vi "niFPGA White Noise Generator.vi"(0 "seed":u32=4294967295, 1 "reset":bool) -> (4 "white noise out":i16)   [LabVIEW 2017]
doc: "Generates a white noise signal with uniform or Gaussian distribution."
uses:
  <vilib>/Platform/TimedLoop/XDataNode/timing_clust.ctl
  <vilib>/Platform/TimedLoop/XDataNode/nitl_modes.ctl
  <vilib>/Platform/TimedLoop/XDataNode/wakeup.ctl
  <vilib>/Platform/TimedLoop/XDataNode/XDataNode.xnode
  <vilib>/Platform/TimedLoop/XDataNode/XDNodeRunTimeDep.lvlib
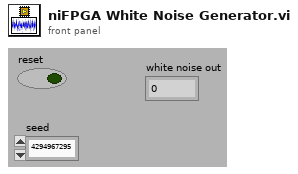
[diagram p1: front panel]
types:
  T1 = typedef "XDNodeRunTimeDep.lvlib/timing_clust.ctl" = cluster{"Expected End [f-1]":u64, "Actual End [f-1]":u64, "Finished Late? [f-1]":bool, "Expected End [i-1]":u64, "Actual End [i-1]":u64, "Finished Late? [i-1]":bool, "Expected Start [i]":u64, "Actual Start [i]":u64, "Expected Start [f]":u64, "Actual Start [f]":u64, "Source Name":string, "Structure Name":string, "Period":i64, "Deadline":i64, "Offset":i64, "Start":i64, "Priority":i32, "Timeout":i32, "Mode":T2, "Wakeup Reason":T3, "Error":errorcluster, "Source Type":string, "Secondary Source Type":string, "Global End Time":u64, "Global Start Time":u64, "Frame Duration":u64, "Iteration Duration":u64, "Assigned CPU":i32, "I/O Scan Engine Mode":u32}
  T2 = typedef "XDNodeRunTimeDep.lvlib/nitl_modes.ctl" = enum32{"No Change", "Process missed periods, maintain original phase", "Discard missed periods, maintain original phase", "Process missed periods, ignore original phase", "Discard missed periods, ignore original phase"}
  T3 = typedef "XDNodeRunTimeDep.lvlib/wakeup.ctl" = enum32{"Normal", "Aborted", "Asynchronous wakeup", "Timing source error", "Timed loop error", "Timeout"}
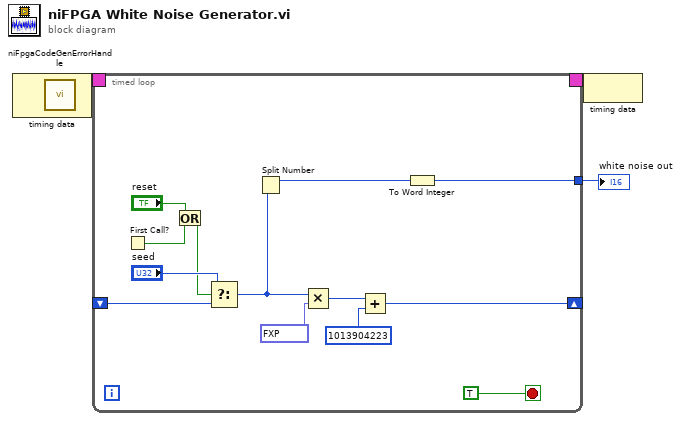
[diagram p0: block diagram]
diagram:
  n1 = node-c288() -> (w3:T1)  [unwired: 1 in]
  n2 = call <vilib>:"niFpgaCodeGenErrorHandle.vi"() -> ()  [unwired: 1 in]
  n3 = timed-loop "Timed Loop" {
    timing: w3 -> [_]
    timing-out: [_] -> w2
    shift-right: [w9] -> _
    shift-left: _ -> [w12]
    tunnel: [w8] -> w1
    stop <- TRUE stop-if-true
    n4 = First Call?() -> (First Call?: T/F=w15:bool)
    n5 = Or(x="reset", y=w15) -> (x .or. y?=w13:bool)
    n6 = Select(t="seed", s=w13, f=w12) -> (s? t:f=w5:u32)
    n7 = Split Number(x=w5) -> (hi(x)=w11:u16)  [unwired: 1 out]
    n8 = Multiply(x=w5, y=fxp<+,21,21> 1664525.0 ("LCG constant A (multiply)")) -> (x*y=w4:u32)
    n9 = Add(x=w4, y=u32 1013904223 ("LCG constant C (add)")) -> (x+y=w9:u32)
    n10 = To Word Integer(number=w11) -> (16bit integer=w8:i16)
  }
  "white noise out" <- w1
  n11 = node-c288(w2) -> ()
